vi "sub_DC Power Middle.vi"(0 "IVI引用句柄输入":refnum<k15>, 1 "instrument handle out":refnum<k15>, 2 "5V":bool, 3 "Source:Output Enabled":bool, 4 "Channel Name 3":string, 5 "错误输入（无错误）":errorcluster, 6 "Channel Name 4":string, 7 "instrument handle out 2":refnum<k15>, 9 "Channel Name 5":string) -> (10 "instrument handle out 3":refnum<k15>, 11 "Current Measurement 2":dbl caption="Current Measurement", 12 "Compliance/Limit Reached":bool, 13 "Voltage Measurement 2":dbl caption="Voltage Measurement" format="%#_3g", 14 "IVI引用句柄输出":refnum<k15>, 15 "Voltage Measurement":dbl format="%#_3g", 17 "Current Measurement":dbl, 18 "Compliance/Limit Reached 2":bool caption="Compliance/Limit Reached", 19 "错误输出":errorcluster)   [LabVIEW 2015]
panel:
  out "Compliance/Limit Reached 3":bool caption="Compliance/Limit Reached"
  out "Current Measurement 3":dbl caption="Current Measurement"
  out "Voltage Measurement 3":dbl caption="Voltage Measurement" format="%#_3g"
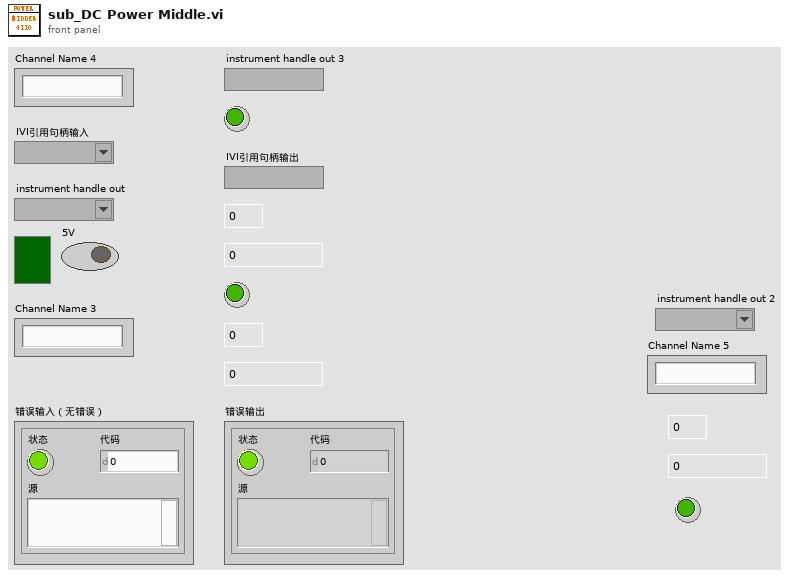
[diagram p1: front panel]
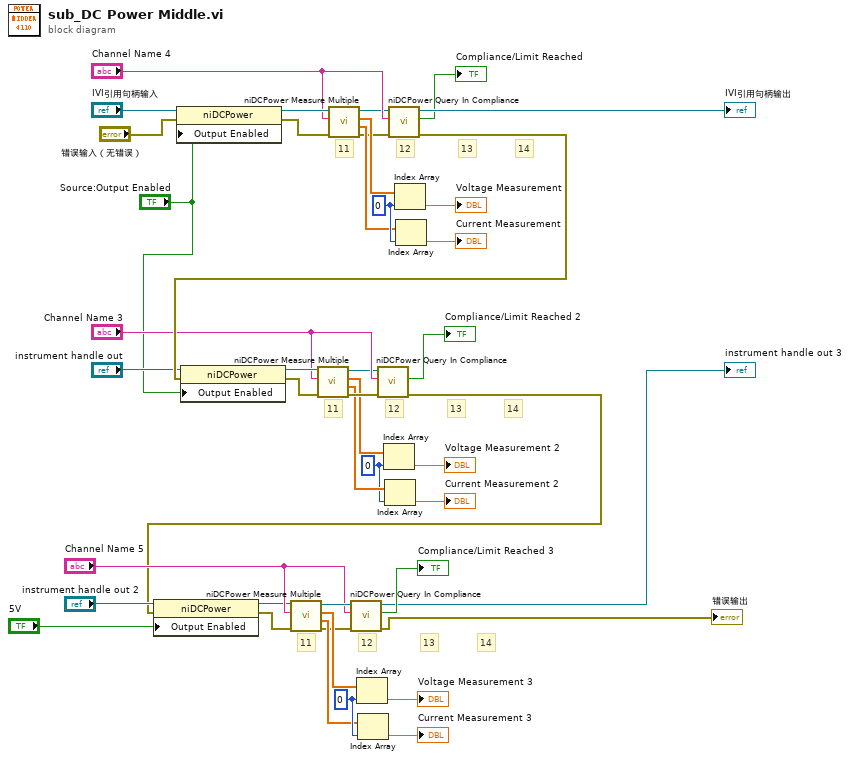
[diagram p0: block diagram]
diagram:
  w14 = 0 ("index")
  w30 = 0 ("index")
  w22 = 0 ("index")
  # "14"
  # "11"
  # "12"
  # "13"
  # "14"
  # "11"
  # "12"
  # "13"
  # "14"
  # "11"
  # "12"
  # "13"
  n1 = property class="niDCPower"(reference="IVI引用句柄输入", error in="错误输入（无错误）", "Output Enabled"="Source:Output Enabled") -> (reference out=w38:refnum<k15>, error out=w39:errorcluster)
  n2 = call <instrlib>:"niDCPower Measure Multiple.vi"("error in (no error)"=w39, "channel name"="Channel Name 4", "instrument handle"=w38) -> ("error out"=w19:errorcluster, "current measurements"=w21:dbl[], "voltage measurements"=w20:dbl[], "instrument handle out"=w18:refnum<k15>)  [unwired: 5 out]
  n3 = call <instrlib>:"niDCPower Query In Compliance.vi"("error in (no error)"=w19, "channel name"="Channel Name 4", "instrument handle"=w18) -> ("error out"=w42:errorcluster, "in compliance?"=→"Compliance/Limit Reached":bool, "instrument handle out"=→"IVI引用句柄输出":refnum<k15>)  [unwired: 6 out]
  n4 = property class="niDCPower"(reference="instrument handle out", error in=w42, "Output Enabled"="Source:Output Enabled") -> (reference out=w43:refnum<k15>, error out=w44:errorcluster)
  n5 = call <instrlib>:"niDCPower Measure Multiple.vi"("error in (no error)"=w44, "channel name"="Channel Name 3", "instrument handle"=w43) -> ("error out"=w33:errorcluster, "current measurements"=w31:dbl[], "voltage measurements"=w32:dbl[], "instrument handle out"=w34:refnum<k15>)  [unwired: 5 out]
  n6 = call <instrlib>:"niDCPower Query In Compliance.vi"("error in (no error)"=w33, "channel name"="Channel Name 3", "instrument handle"=w34) -> ("error out"=w5:errorcluster, "in compliance?"=→"Compliance/Limit Reached 2":bool)  [unwired: 7 out]
  n7 = property class="niDCPower"(reference="instrument handle out 2", error in=w5, "Output Enabled"="5V") -> (reference out=w7:refnum<k15>, error out=w6:errorcluster)
  n8 = call <instrlib>:"niDCPower Measure Multiple.vi"("error in (no error)"=w6, "channel name"="Channel Name 5", "instrument handle"=w7) -> ("error out"=w11:errorcluster, "current measurements"=w13:dbl[], "voltage measurements"=w12:dbl[], "instrument handle out"=w10:refnum<k15>)  [unwired: 5 out]
  n9 = call <instrlib>:"niDCPower Query In Compliance.vi"("error in (no error)"=w11, "channel name"="Channel Name 5", "instrument handle"=w10) -> ("error out"=→"错误输出":errorcluster, "in compliance?"=→"Compliance/Limit Reached 3":bool, "instrument handle out"=→"instrument handle out 3":refnum<k15>)  [unwired: 6 out]
  n10 = Index Array(array=w12, index=w14) -> (element=→"Voltage Measurement 3":dbl)
  n11 = Index Array(array=w13, index=w14) -> (element=→"Current Measurement 3":dbl)
  n12 = Index Array(array=w32, index=w30) -> (element=→"Voltage Measurement 2":dbl)
  n13 = Index Array(array=w31, index=w30) -> (element=→"Current Measurement 2":dbl)
  n14 = Index Array(array=w20, index=w22) -> (element=→"Voltage Measurement":dbl)
  n15 = Index Array(array=w21, index=w22) -> (element=→"Current Measurement":dbl)
